vi "Controller Monitoring Loop.vi"(7 "Sync Objects":T1, 8 "error in (no error)":errorcluster, 11 "FOFB Configuration":T5={"FOFB Parameters"={"Network"={"FOFB Controller IP"="", "LNLS Control Network IP"="", "LNLS Control Network Power Supplies TCP Port"=0, "LNLS Control Network FOFB Configuration TCP Port"=0, "Data Server TCP Port"=0, "Monitoring Data TCP Port"=0, "Configuration GUI TCP Port"=0, "TCP Listening Timeout"=0}, "Fast Acquisition"={"Acquisition Period"=0, "Data Buffer Size"=0}, "Response Matrix Measurement"={"Step Amplitude"=0.0, "Time Between Steps"=0, "Step Duration"=0, "Number of Averages"=0}, "Correction Algorithm"={"Correction Period"=0, "Reference Orbit Path"=path "", "Response Matrix Path"=path "", "Correction Matrix Path"=path "", "Horizontal Correction Factor"=0.0, "Vertical Correction Factor"=0.0, "Beam Current FOFB Threshold"=0.0, "Decouple H-V"=FALSE}, "Acquisition Network"=[], "Actuation Network"=[]}, "Number of Acquisition Chassis"=0, "Number of Actuation Chassis"=0, "Number of BPM Readings"=0, "BPM Reading Names"=[], "Selected BPM Readings"=[0, 1, 2, 3, 4, 5, 6, 7, 8, 9, 10, 11, 12, 13, 14, 15, 16, 17, 18, 19, 20, 21, 22, 23, 24, 25, 26, 27, 28, 29, 30, 31, 32, 33, 34, 35, 36, 37, 38, 39, 40, 41, 42, 43, 44, 45, 46, 47, 48, 49], "Number of Correctors"=0, "Corrector Names"=[], "Selected Correctors"=[0, 1, 2, 3, 4, 5, 6, 7, 8, 9, 10, 11, 12, 13, 14, 15, 16, 17, 18, 19, 20, 21, 22, 23, 24, 25, 26, 27, 28, 29, 30, 31, 32, 33, 34, 35, 36, 37, 38, 39, 40, 41, 42, 43, 44, 45, 46, 47, 48, 49], "Reference Orbit"=[], "Response Matrix"=[], "Correction Matrix"=[], "Acquisition Chassis Names"=[], "Actuation Chassis Names"=[], "Acquisition Variables"=[], "Actuation Variables"=[], "PS Matrix Mapping"=[], "Inverse PS Matrix Mapping"=[], "Response Matrix Beam Energy (MeV)"=0.0, "PID Parameters"=[], "BPM Planes"=[], "Corrector Planes"=[], "RMM Step Factor"=[]}) -> (0 "error out":errorcluster)   [LabVIEW 2011, in "Controller VIs.lvlib"]
uses:
  Controller VIs.lvlib
  Types Definitions/Type FOFB Configuration.ctl
  Types Definitions/Type FOFB Parameters.ctl
  Types Definitions/Type Network Configuration.ctl
  Types Definitions/Type FA Configuration.ctl
  Types Definitions/Type Response Matrix Measurement Configuration.ctl
  Types Definitions/Type Correction Algorithm Configuration.ctl
  Types Definitions/Type Acquisition Network Configuration.ctl
  Types Definitions/Type Actuation Network Configuration.ctl
  Types Definitions/Type PID Parameters.ctl
  Types Definitions/Type Synchronization Objects.ctl
  Types Definitions/Type Blocking Synchronization Objects.ctl
  Types Definitions/Type FA Request Parameters.ctl
  Types Definitions/Type BPM and PS select cluster.ctl
  Types Definitions/Type FA File Parameters.ctl
  Types Definitions/Type Monitoring Data.ctl
  Types Definitions/Type Diagnostics Data.ctl
  Types Definitions/Type CPU Loads Array.ctl
  Types Definitions/Type CPU Loads.ctl
  Types Definitions/Type Non-blocking Synchronization Objects.ctl
  Types Definitions/Type FOFB Variables.ctl
  Types Definitions/Type Actuation State.ctl
  <vilib>/Platform/TimedLoop/XDataNode/timing_clust.ctl
  <vilib>/Platform/TimedLoop/XDataNode/nitl_modes.ctl
  <vilib>/Platform/TimedLoop/XDataNode/wakeup.ctl
  Controller Global Variables/Controller Operation Mode.vi
  Controller Global Variables/Controller Status Table.vi
  Controller Global Variables/Monitoring Data.vi
  <vilib>/Platform/TimedLoop/XDataNode/XDataNode.xnode
  Filter VIs.lvlib
  Type Definitions.lvlib
  <vilib>/NI_Real-Time Target Support.lvlib
  Controller Global Variables.lvlib
  <vilib>/Platform/TimedLoop/XDataNode/XDNodeRunTimeDep.lvlib
panel:
  out "Monitoring Data Period (ms)":dbl
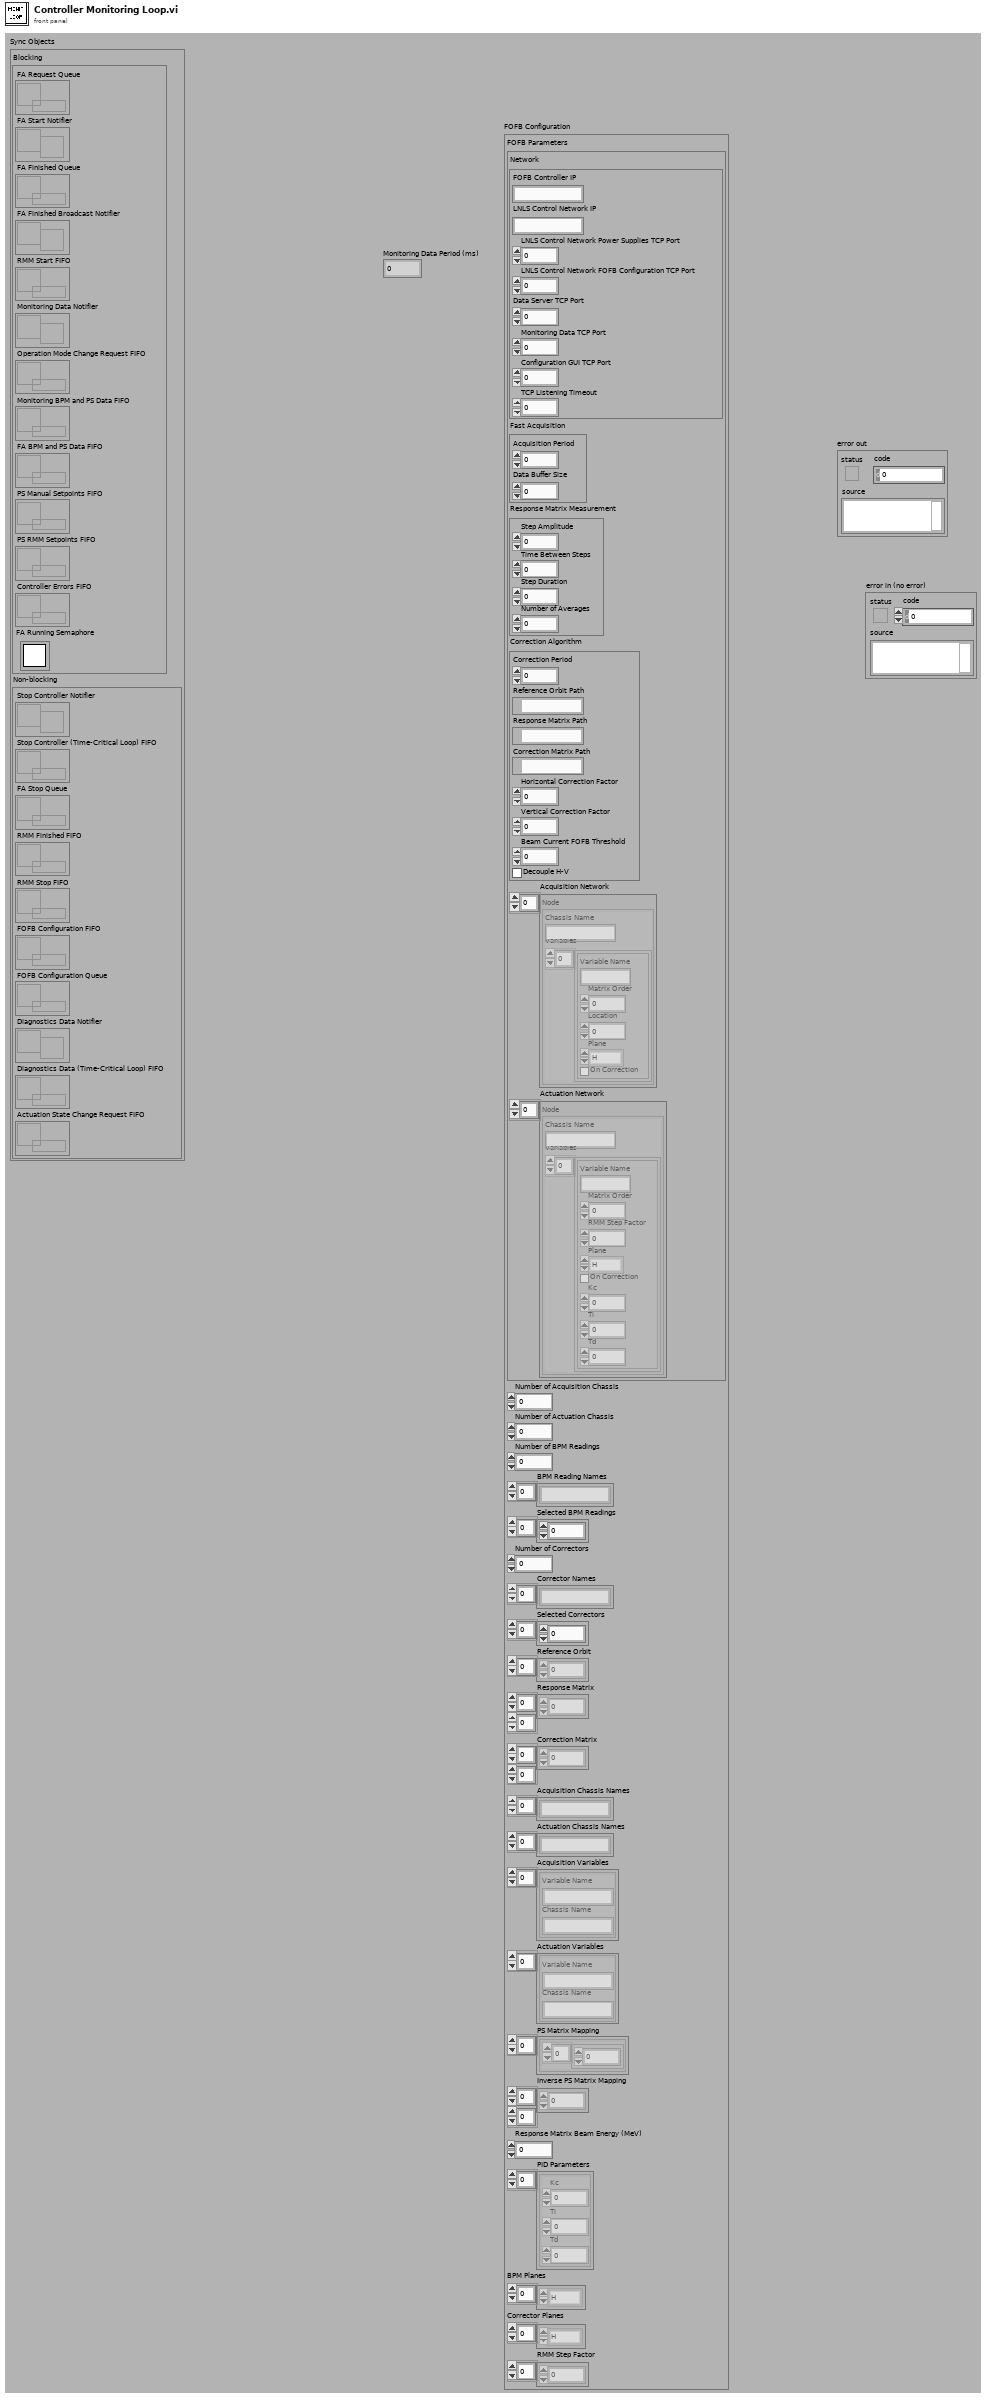
[diagram p1: front panel]
types:
  T1 = typedef "Type Definitions.lvlib/Type Synchronization Objects.ctl" = cluster{"Blocking":T2, "Non-blocking":T4}
  T2 = typedef "Type Definitions.lvlib/Type Blocking Synchronization Objects.ctl" = cluster{"FA Request Queue":refnum<queue>, "FA Start Notifier":refnum<notifier>, "FA Finished Queue":refnum<queue>, "FA Finished Broadcast Notifier":refnum<notifier>, "RMM Start FIFO":refnum<k33>, "Monitoring Data Notifier":refnum<notifier>, "Operation Mode Change Request FIFO":refnum<k33>, "Monitoring BPM and PS Data FIFO":refnum<k33>, "FA BPM and PS Data FIFO":refnum<k33>, "PS Manual Setpoints FIFO":refnum<k33>, "PS RMM Setpoints FIFO":refnum<k33>, "Controller Errors FIFO":refnum<k33>, "FA Running Semaphore":T3}
  T3 = typedef "Semaphore RefNum" = refnum<k1>
  T4 = typedef "Type Definitions.lvlib/Type Non-blocking Synchronization Objects.ctl" = cluster{"Stop Controller Notifier":refnum<notifier>, "Stop Controller (Time-Critical Loop) FIFO":refnum<k33>, "FA Stop Queue":refnum<queue>, "RMM Finished FIFO":refnum<k33>, "RMM Stop FIFO":refnum<k33>, "FOFB Configuration FIFO":refnum<k33>, "FOFB Configuration Queue":refnum<queue>, "Diagnostics Data Notifier":refnum<notifier>, "Diagnostics Data (Time-Critical Loop) FIFO":refnum<k33>, "Actuation State Change Request FIFO":refnum<k33>}
  T5 = typedef "Type Definitions.lvlib/Type FOFB Configuration.ctl" = cluster{"FOFB Parameters":T6, "Number of Acquisition Chassis":i32, "Number of Actuation Chassis":i32, "Number of BPM Readings":i32, "BPM Reading Names":string[], "Selected BPM Readings":u32[], "Number of Correctors":i32, "Corrector Names":string[], "Selected Correctors":u32[], "Reference Orbit":dbl[], "Response Matrix":dbl[][], "Correction Matrix":dbl[][], "Acquisition Chassis Names":string[], "Actuation Chassis Names":string[], "Acquisition Variables":cluster{"Variable Name":string, "Chassis Name":string}[], "Actuation Variables":cluster{"Variable Name":string, "Chassis Name":string}[], "PS Matrix Mapping":cluster{u32[]}[], "Inverse PS Matrix Mapping":u32[][], "Response Matrix Beam Energy (MeV)":dbl, "PID Parameters":T13[], "BPM Planes":enum8{"H", "V"}[], "Corrector Planes":enum8{"H", "V"}[], "RMM Step Factor":dbl[]}
  T6 = typedef "Type Definitions.lvlib/Type FOFB Parameters.ctl" = cluster{"Network":T7, "Fast Acquisition":T8, "Response Matrix Measurement":T9, "Correction Algorithm":T10, "Acquisition Network":T11, "Actuation Network":T12}
  T7 = typedef "Type Definitions.lvlib/Type Network Configuration.ctl" = cluster{"FOFB Controller IP":string, "LNLS Control Network IP":string, "LNLS Control Network Power Supplies TCP Port":u16, "LNLS Control Network FOFB Configuration TCP Port":u16, "Data Server TCP Port":u16, "Monitoring Data TCP Port":u16, "Configuration GUI TCP Port":u16, "TCP Listening Timeout":i32}
  T8 = typedef "Type Definitions.lvlib/Type FA Configuration.ctl" = cluster{"Acquisition Period":u32, "Data Buffer Size":u32}
  T9 = typedef "Type Definitions.lvlib/Type Response Matrix Measurement Configuration.ctl" = cluster{"Step Amplitude":dbl, "Time Between Steps":u32, "Step Duration":u32, "Number of Averages":u32}
  T10 = typedef "Type Definitions.lvlib/Type Correction Algorithm Configuration.ctl" = cluster{"Correction Period":u32, "Reference Orbit Path":path, "Response Matrix Path":path, "Correction Matrix Path":path, "Horizontal Correction Factor":dbl, "Vertical Correction Factor":dbl, "Beam Current FOFB Threshold":dbl, "Decouple H-V":bool}
  T11 = typedef "Type Definitions.lvlib/Type Acquisition Network Configuration.ctl" = cluster{"Chassis Name":string, "Variables":cluster{"Variable Name":string, "Matrix Order":u32, "Location":dbl, "Plane":enum8{"H", "V"}, "On Correction":bool}[]}[]
  T12 = typedef "Type Definitions.lvlib/Type Actuation Network Configuration.ctl" = cluster{"Chassis Name":string, "Variables":cluster{"Variable Name":string, "Matrix Order":u32, "RMM Step Factor":dbl, "Plane":enum8{"H", "V"}, "On Correction":bool, "Kc":dbl, "Ti":dbl, "Td":dbl}[]}[]
  T13 = typedef "Type Definitions.lvlib/Type PID Parameters.ctl" = cluster{"Kc":fxp<+/-,16,8>, "Ti":fxp<+/-,16,8>, "Td":fxp<+/-,16,8>}
  T14 = enum16{"Idle", "Wait Connection", "Write Data", "Close Connection"}
  T15 = typedef "XDNodeRunTimeDep.lvlib/timing_clust.ctl" = cluster{"Expected End [f-1]":u64, "Actual End [f-1]":u64, "Finished Late? [f-1]":bool, "Expected End [i-1]":u64, "Actual End [i-1]":u64, "Finished Late? [i-1]":bool, "Expected Start [i]":u64, "Actual Start [i]":u64, "Expected Start [f]":u64, "Actual Start [f]":u64, "Source Name":string, "Structure Name":string, "Period":i64, "Deadline":i64, "Offset":i64, "Start":i64, "Priority":i32, "Timeout":i32, "Mode":T16, "Wakeup Reason":T17, "Error":errorcluster, "Source Type":string, "Secondary Source Type":string, "Global End Time":u64, "Global Start Time":u64, "Frame Duration":u64, "Iteration Duration":u64, "Assigned CPU":i32, "I/O Scan Engine Mode":u32}
  T16 = typedef "XDNodeRunTimeDep.lvlib/nitl_modes.ctl" = enum32{"No Change", "Process missed periods, maintain original phase", "Discard missed periods, maintain original phase", "Process missed periods, ignore original phase", "Discard missed periods, ignore original phase"}
  T17 = typedef "XDNodeRunTimeDep.lvlib/wakeup.ctl" = enum32{"Normal", "Aborted", "Asynchronous wakeup", "Timing source error", "Timed loop error", "Timeout"}
  T18 = typedef "Type Definitions.lvlib/Type Monitoring Data.ctl" = cluster{"Timestamp":timestamp, "BPM Readings":dbl[], "PS Readings":dbl[], "PS FOFB Setpoints":dbl[], "PS Status per Rack":u8[], "PS ON-OFF per Rack":u8[], "Operation Mode":enum16{"Idle Mode", "Error Mode", "Manual Mode", "FOFB Mode", "RMM Mode"}, "Diagnostics Data":T19, "Controller Status Table":i32[]}
  T19 = typedef "Type Definitions.lvlib/Type Diagnostics Data.ctl" = cluster{"Time-Critical Loop Missed Iterations":u32, "Time-Critical Loop Execution Time (usec)":u32, "FA Buffer Usage":u32, "Available Memory (bytes)":u32, "CPU Loads Array":T20}
  T20 = typedef "Type Definitions.lvlib/Type CPU Loads Array.ctl" = T21[]
  T21 = typedef "Type Definitions.lvlib/Type CPU Loads.ctl" = cluster{"Total (%)":dbl, "Time Critical (%)":dbl, "Timed Structures (%)":dbl, "High (%)":dbl, "Above Normal (%)":dbl, "Normal (%)":dbl, "Background (%)":dbl, "Idle (%)":dbl, "ISR (%)":dbl}
  T22 = typedef "Type Definitions.lvlib/Type FA File Parameters.ctl" = cluster{"FA Parameters":T23, "File Reference":refnum<file>}
  T23 = typedef "Type Definitions.lvlib/Type FA Request Parameters.ctl" = cluster{"Number of Samples":u32, "BPM and PS Selection":T24, "Filename":string}
  T24 = typedef "Type Definitions.lvlib/Type BPM and PS select cluster.ctl" = cluster{"BPM index array":u32[], "PS index array ":u32[]}
  T25 = typedef "NI_Real-Time Target Support.lvlib/RT CPU Load.ctl" = cluster{"Total (%)":dbl, "Time Critical (%)":dbl, "Timed Structures (%)":dbl, "High (%)":dbl, "Above Normal (%)":dbl, "Normal (%)":dbl, "Background (%)":dbl, "Idle (%)":dbl, "ISR (%)":dbl}
  T26 = enum16{"Idle Mode", "Error Mode", "Manual Mode", "FOFB Mode", "RMM Mode"}
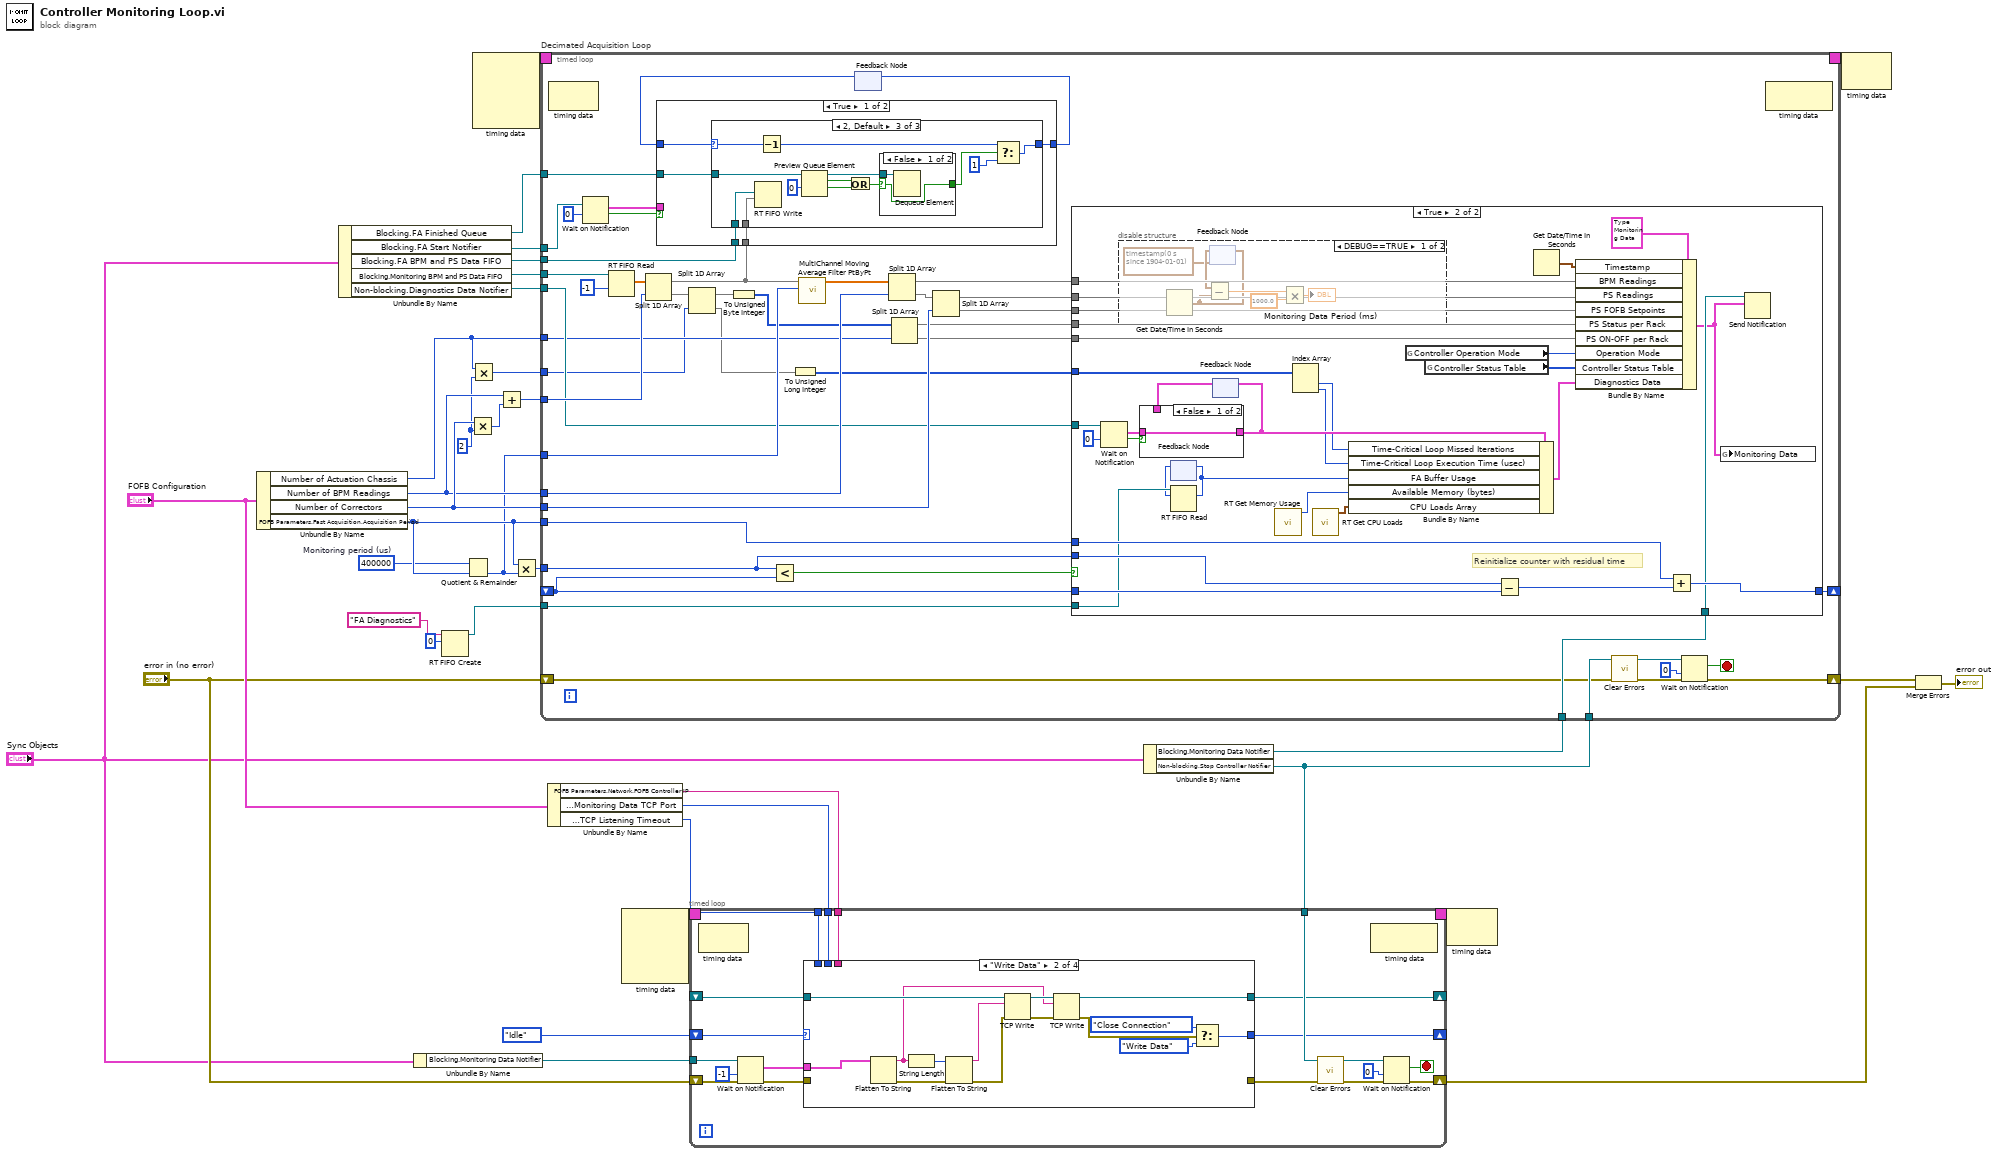
[diagram p0: block diagram]
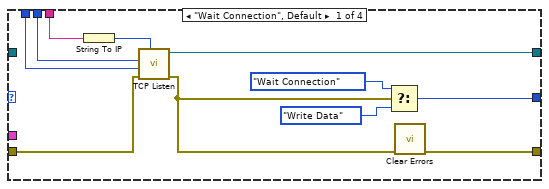
[diagram p2: hidden frame]
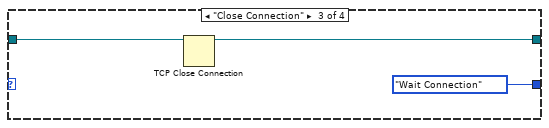
[diagram p3: hidden frame]
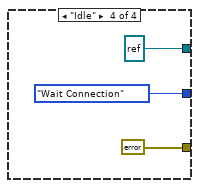
[diagram p4: hidden frame]
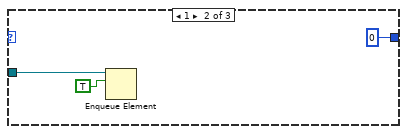
[diagram p6: hidden frame]
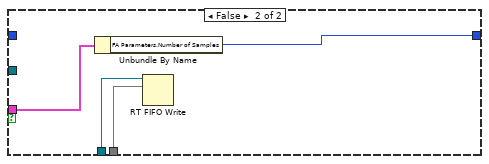
[diagram p8: hidden frame]
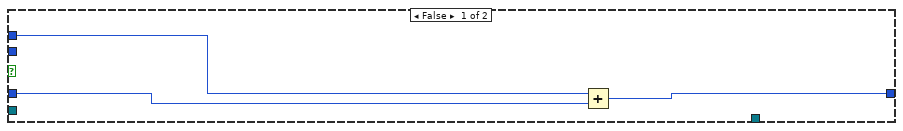
[diagram p9: hidden frame]
diagram:
  w9 = u32 400000  # Monitoring period (us)
  w13 = 2 ("y")
  n1 = Unbundle By Name("FOFB Configuration") -> ("Number of Actuation Chassis"=w12:i32, "Number of BPM Readings"=w20:i32, "Number of Correctors"=w21:i32, "FOFB Parameters.Fast Acquisition.Acquisition Period"=w10:u32)
  n2 = Unbundle By Name("Sync Objects") -> ("Blocking.FA Finished Queue"=w14:refnum<queue>, "Blocking.FA Start Notifier"=w15:refnum<notifier>, "Blocking.FA BPM and PS Data FIFO"=w16:refnum<k33>, "Blocking.Monitoring BPM and PS Data FIFO"=w22:refnum<k33>, "Non-blocking.Diagnostics Data Notifier"=w17:refnum<notifier>)
  n3 = Unbundle By Name("Sync Objects") -> ("Blocking.Monitoring Data Notifier"=w27:refnum<notifier>)
  n4 = RT FIFO Create(0:"FA Diagnostics" ("name (unnamed)"), 1:0 ("# elements")) -> (8:w1:refnum<k33>)  [unwired: 6 in, 2 out]
  n5 = Quotient & Remainder(x=w9, y=w10) -> (floor(x/y)=w8:u32)  [unwired: 1 out]
  n6 = Multiply(x=w21, y=w13) -> (x*y=w19:i32)
  n7 = Multiply(x=w12, y=w13) -> (x*y=w11:i32)
  n8 = node-c288() -> (w7:T15)  [unwired: 4 in]
  n9 = Add(x=w20, y=w19) -> (x+y=w18:i32)
  n10 = Multiply(x=w10, y=w8) -> (x*y=w24:u32)
  n11 = Unbundle By Name("FOFB Configuration") -> ("FOFB Parameters.Network.FOFB Controller IP"=w35:string, "FOFB Parameters.Network.Monitoring Data TCP Port"=w28:u16, "FOFB Parameters.Network.TCP Listening Timeout"=w34:i32)
  n12 = node-c288() -> (w5:T15)  [unwired: 4 in]
  n13 = Unbundle By Name("Sync Objects") -> ("Blocking.Monitoring Data Notifier"=w26:refnum<notifier>, "Non-blocking.Stop Controller Notifier"=w32:refnum<notifier>)
  n14 = timed-loop "Decimated Acquisition Loop" {
    shift-right: [w78] -> w31
    shift-left: "error in (no error)" -> [w56]
    tunnel: w32 -> [w76]
    tunnel: w20 -> [w70]
    tunnel: w21 -> [w69]
    tunnel: w10 -> [w68]
    tunnel: w24 -> [w67]
    tunnel: w26 -> [w65]
    tunnel: w8 -> [w64]
    shift-right: [w62] -> _
    shift-left: _ -> [w63]
    tunnel: w22 -> [w60]
    tunnel: w18 -> [w58]
    tunnel: w17 -> [w57]
    tunnel: w16 -> [w55]
    tunnel: w15 -> [w52]
    tunnel: w14 -> [w49]
    tunnel: w12 -> [w45]
    tunnel: w11 -> [w42]
    timing: w7 -> [_]
    timing-out: [_] -> w6
    tunnel: w1 -> [w39]
    stop <- w77 stop-if-true
    n15 = node-c288() -> ()  [unwired: 1 in, 1 out]
    n16 = Wait on Notification(notifier=w52, timeout in ms (-1)=0) -> (notification=w38:T22, timed out?=w37:bool)  [unwired: 2 in, 2 out]
    n17 = RT FIFO Read(0:w60, 2:-1 ("timeout in ms (0)")) -> (9:w59:dbl[])  [unwired: 2 in, 4 out]
    n18 = Split 1D Array(array=w59, index=w58) -> (first subarray=w54:dbl[], second subarray=w44:dbl[])
    n19 = Split 1D Array(array=w44, index=w42) -> (first subarray=w43:dbl[], second subarray=w40:dbl[])
    n20 = To Unsigned Byte Integer(number=w43) -> (unsigned 8bit integer=w48:u8[])
    n21 = Less?(x=w67, y=w63) -> (x < y?=w66:bool)
    n22 = To Unsigned Long Integer(number=w40) -> (unsigned 32bit integer=w41:u32[])
    n23 = call "MultiChannel Moving Average Filter PtByPt.vi"("Number of Averages"=w64, "X"=w54) -> ("Filtered X"=w75:dbl[])  [unwired: 9 in]
    n24 = feedback #1() -> (w50:u32)  [unwired: 1 in]
    n25 = case shown="True" w37 {
      tunnel: w55 -> [w87 w111]
      tunnel: w54 -> [w86 w110]
      tunnel: w38 -> [_ w108]
      tunnel: [w85 w109] -> w51
      tunnel: w50 -> [w83 _]
      tunnel: w49 -> [w84 _]
      frame True {
        n26 = case shown="2, Default" w83 {
          selector: w83 -> [w88 _ w93]
          tunnel: w87 -> [_ _ w104]
          tunnel: w86 -> [_ _ w103]
          tunnel: [w88 u32 0 ("f") w100] -> w85
          tunnel: w84 -> [_ w90 w101]
          frame 0 {
          }
          frame 1 {
            n27 = Enqueue Element(queue=w90, element=TRUE) -> ()  [unwired: 2 in, 3 out]
          }
          frame 2, Default {
            n28 = RT FIFO Write(0:w104, 1:w103) -> ()  [unwired: 3 in, 4 out]
            n29 = Decrement(x=w93) -> (x-1=w92:u32)
            n30 = Preview Queue Element(queue=w101, timeout in ms (-1)=0) -> (queue out=w98:refnum<queue>, element=w97:bool, timed out?=w96:bool)  [unwired: 1 in, 1 out]
            n31 = Or(x=w97, y=w96) -> (x .or. y?=w95:bool)
            n32 = case shown="False" w95 {
              selector: w95 -> [w105 w107]
              tunnel: w98 -> [w106 _]
              tunnel: [w105 w107] -> w94
              frame False {
                n33 = Dequeue Element(queue=w106) -> ()  [unwired: 2 in, 4 out]
              }
              frame True {
              }
            }
            n34 = Select(t=w92, s=w94, f=u32 1) -> (s? t:f=w100:u32)
          }
        }
      }
      frame False {
        n35 = Unbundle By Name(w108) -> ("FA Parameters.Number of Samples"=w109:u32)
        n36 = RT FIFO Write(0:w111, 1:w110) -> ()  [unwired: 3 in, 4 out]
      }
    }
    n37 = feedback-in #1(w51) -> ()
    n38 = Split 1D Array(array=w75, index=w70) -> (first subarray=w74:dbl[], second subarray=w73:dbl[])
    n39 = Split 1D Array(array=w48, index=w45) -> (first subarray=w47:u8[], second subarray=w46:u8[])
    n40 = Split 1D Array(array=w73, index=w69) -> (first subarray=w72:dbl[], second subarray=w71:dbl[])
    n41 = case shown="True" w66 {
      tunnel: w74 -> [_ w139]
      tunnel: w72 -> [_ w138]
      tunnel: w71 -> [_ w137]
      tunnel: [w112 w144] -> w62
      tunnel: w63 -> [w113 w143]
      tunnel: w67 -> [_ w142]
      tunnel: w68 -> [w114 w141]
      tunnel: w65 -> [_ w135]
      tunnel: w47 -> [_ w131]
      tunnel: w57 -> [_ w125]
      tunnel: w46 -> [_ w122]
      tunnel: w41 -> [_ w121]
      tunnel: w39 -> [_ w117]
      frame False {
        n42 = Add(x=w114, y=w113) -> (x+y=w112:u32)
      }
      frame True {
        # "Reinitialize counter with residual time"
        n43 = Wait on Notification(notifier=w125, timeout in ms (-1)=0) -> (notification=w127:T19, timed out?=w128:bool)  [unwired: 2 in, 2 out]
        n44 = disable-structure shown="DEBUG==TRUE" {
          frame condition #0 {
            n45 = Get Date/Time In Seconds() -> (seconds since 1Jan1904=w146:timestamp)
            n46 = feedback #2(timestamp(0 s since 1904-01-01)) -> (w151:timestamp)
            n47 = Subtract(x=w151, y=w146) -> (x-y=w149:dbl)
            n48 = feedback-in #2(w146) -> ()
            n49 = Multiply(x=w149, y=1000.0) -> (x*y=→"Monitoring Data Period (ms)":dbl)
          }
          frame condition #1 (active) {
          }
        }
        n50 = feedback #3() -> (w116:i32)  [unwired: 1 in]
        n51 = RT FIFO Read(0:w117, 1:w116) -> (9:w115:i32)  [unwired: 2 in, 4 out]
        n52 = feedback-in #3(w115) -> ()
        n53 = feedback #4() -> (w129:T19)  [unwired: 1 in]
        n54 = case shown="False" w128 {
          tunnel: [w152 w153] -> w126
          tunnel: w127 -> [w152 _]
          tunnel: w129 -> [_ w153]
          frame False {
          }
          frame True {
          }
        }
        n55 = feedback-in #4(w126) -> ()
        n56 = call <vilib>:"RT Get Memory Usage.vi"() -> ("total (bytes)"=w118:u32)  [unwired: 8 in, 3 out]
        n57 = Index Array(array=w121) -> (element #1=w120:u32, element #2=w119:u32)  [unwired: 2 in]
        n58 = call <vilib>:"RT Get CPU Loads.vi"() -> ("CPU loads"=w134:T25[])  [unwired: 10 in, 1 out]
        n59 = Bundle By Name(cluster=w126, "Time-Critical Loop Missed Iterations"=w120, "Time-Critical Loop Execution Time (usec)"=w119, "FA Buffer Usage"=w115, "Available Memory (bytes)"=w118, "CPU Loads Array"=w134) -> (w133:T19)
        n60 = global read "Controller Operation Mode.vi" "Controller Operation Mode"() -> (w123:T26)
        n61 = global read "Controller Status Table.vi" "Controller Status Table"() -> (w124:i32[])
        n62 = Subtract(x=w142, y=w143) -> (x-y=w145:u32)
        n63 = Get Date/Time In Seconds() -> (seconds since 1Jan1904=w140:timestamp)
        n64 = Bundle By Name(cluster=T18 {"Timestamp"=timestamp(0 s since 1904-01-01), "BPM Readings"=[], "PS Readings"=[], "PS FOFB Setpoints"=[], "PS Status per Rack"=[], "PS ON-OFF per Rack"=[], "Operation Mode"=enum."Idle Mode", "Diagnostics Data"={"Time-Critical Loop Missed Iterations"=0, "Time-Critical Loop Execution Time (usec)"=0, "FA Buffer Usage"=0, "Available Memory (bytes)"=0, "CPU Loads Array"=[]}, "Controller Status Table"=[]} ("output cluster"), "Timestamp"=w140, "BPM Readings"=w139, "PS Readings"=w138, "PS FOFB Setpoints"=w137, "PS Status per Rack"=w131, "PS ON-OFF per Rack"=w122, "Operation Mode"=w123, "Controller Status Table"=w124, "Diagnostics Data"=w133) -> (w132:T18)
        n65 = Add(x=w141, y=w145) -> (x+y=w144:u32)
        n66 = global write "Monitoring Data.vi" "Monitoring Data"(w132) -> ()
        n67 = Send Notification(notification=w132, notifier=w135) -> ()  [unwired: 1 in, 2 out]
      }
    }
    n68 = call <vilib>:"Clear Errors.vi"("error in (no error)"=w56) -> ("error out"=w79:errorcluster)  [unwired: 6 in]
    n69 = Wait on Notification(notifier=w76, timeout in ms (-1)=0, error in (no error)=w79) -> (notification=w77:bool, error out=w78:errorcluster)  [unwired: 1 in, 2 out]
    n70 = node-c288() -> ()  [unwired: 1 in, 1 out]
  }
  n71 = timed-loop {
    tunnel: w35 -> [w171]
    tunnel: w28 -> [w170]
    tunnel: w34 -> [w169]
    shift-right: [w166] -> w30
    shift-left: "error in (no error)" -> [w162]
    tunnel: w32 -> [w165]
    tunnel: w27 -> [w164]
    shift-right: [w160] -> _
    shift-left: T14."Idle" ("f") -> [w161]
    shift-right: [w158] -> _
    shift-left: _ -> [w159]
    timing: w5 -> [_]
    timing-out: [_] -> w4
    stop <- w167 stop-if-true
    # "ms"
    n72 = node-c288() -> ()  [unwired: 1 in, 1 out]
    n73 = Wait on Notification(notifier=w164, timeout in ms (-1)=-1, error in (no error)=w162) -> (notification=w163:T18, error out=w156:errorcluster)  [unwired: 1 in, 2 out]
    n74 = case shown="\"Write Data\"" w161 {
      tunnel: [w184 w198 w201 refnum<k5> refnum ("connection ID")] -> w158
      tunnel: [w183 w197 T14."Wait Connection" ("f") T14."Wait Connection" ("f")] -> w160
      tunnel: [w181 _ _ errorcluster {"status"=FALSE, "code"=0, "source"=""} ("error out")] -> w155
      tunnel: w156 -> [w178 _ _ _]
      tunnel: w159 -> [_ w192 w199 _]
      tunnel: w171 -> [w177 _ _ _]
      tunnel: w170 -> [w175 _ _ _]
      tunnel: w169 -> [w174 _ _ _]
      tunnel: w163 -> [_ w187 _ _]
      frame "Wait Connection", Default {
        n75 = String To IP(1:w177) -> (0:w176:u32)
        n76 = call <vilib>:"TCP Listen.vi"("net address"=w176, "error in (no error)"=w178, "timeout ms (wait forever: -1)"=w174, "port"=w175) -> ("error out"=w182:errorcluster, "connection ID"=w184:refnum<k5>)  [unwired: 3 in, 3 out]
        n77 = Select(t=T14."Wait Connection" ("f"), s=w182, f=T14."Write Data") -> (s? t:f=w183:T14)
        n78 = call <vilib>:"Clear Errors.vi"("error in (no error)"=w182) -> ("error out"=w181:errorcluster)  [unwired: 6 out]
      }
      frame "Write Data" {
        n79 = Flatten To String(anything=w187) -> (data string=w188:string, error out=w186:errorcluster)  [unwired: 3 in, 1 out]
        n80 = String Length(string=w188) -> (length=w190:i32)
        n81 = Flatten To String(anything=w190, error in (no error)=w186) -> (data string=w189:string, error out=w185:errorcluster)  [unwired: 2 in, 1 out]
        n82 = TCP Write(connection ID=w192, data in=w189, error in (no error)=w185) -> (connection ID out=w193:refnum<k5>, error out=w191:errorcluster)  [unwired: 2 out]
        n83 = TCP Write(connection ID=w193, data in=w188, error in (no error)=w191) -> (connection ID out=w198:refnum<k5>, error out=w196:errorcluster)  [unwired: 2 out]
        n84 = Select(t=T14."Close Connection" ("f"), s=w196, f=T14."Write Data") -> (s? t:f=w197:T14)
      }
      frame "Close Connection" {
        n85 = TCP Close Connection(connection ID=w199) -> (connection ID out=w201:refnum<k5>)  [unwired: 2 in, 1 out]
      }
      frame "Idle" {
      }
    }
    n86 = call <vilib>:"Clear Errors.vi"("error in (no error)"=w155) -> ("error out"=w154:errorcluster)  [unwired: 6 in]
    n87 = node-c288() -> ()  [unwired: 1 in, 1 out]
    n88 = Wait on Notification(notifier=w165, timeout in ms (-1)=0, error in (no error)=w154) -> (notification=w167:bool, error out=w166:errorcluster)  [unwired: 1 in, 2 out]
  }
  n89 = node-c288(w4) -> ()  [unwired: 1 out]
  n90 = node-c288(w6) -> ()  [unwired: 1 out]
  n91 = Merge Errors(w31, w30) -> (→"error out":errorcluster)
